vi "Report Invalid Receiver.vi"(8 "Error In":errorcluster, 10 "Receiver":string, 11 "Central Message Handler In":refnum<class "Central Message Handler.lvclass">) -> (0 "Error Out":errorcluster, 3 "Central Message Handler Out":refnum<class "Central Message Handler.lvclass">)   [LabVIEW 2019, in "Central Message Handler.lvclass"]
uses:
  Central Message Handler.lvclass
  Process/Public/Controls/Process Message.ctl
  <vilib>/Utility/error.llb/Error Cluster From Error Code.vi
  <vilib>/ErrorRing/Error Ring.xnode
  Process/Process.lvclass
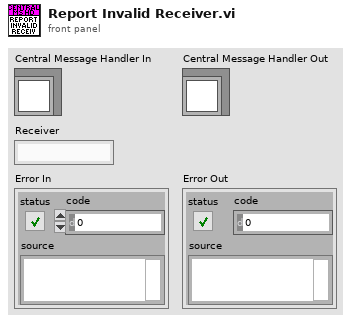
[diagram p1: front panel]
types:
  T1 = typedef "Process.lvclass/Process Message.ctl" = cluster{"Command":string, "Data":variant}
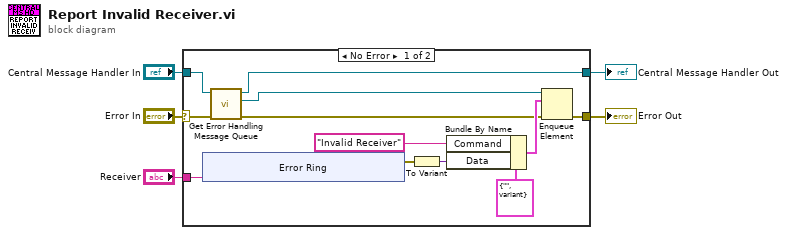
[diagram p0: block diagram]
diagram:
  n1 = case shown="No Error" "Error In" {
    selector: "Error In" -> [w10 w25]
    tunnel: "Receiver" -> [w17 _]
    tunnel: [w16 w25] -> w4
    tunnel: "Central Message Handler In" -> [w11 w26]
    tunnel: [w8 w26] -> w1
    frame No Error {
      n2 = xnode "Error Ring"("parameter 0"=w17) -> ("error out"=w6:errorcluster)
      n3 = call "Get Error Handling Message Queue.vi"("Error In"=w10, "Central Message Handler In"=w11) -> ("Error Out"=w9:errorcluster, "Error Handling Message Queue"=w14:refnum<queue>, "Central Message Handler Out"=w8:refnum<class "Central Message Handler.lvclass">)  [unwired: 7 in]
      n4 = To Variant(anything=w6) -> (Variant=w7:variant)
      n5 = Bundle By Name(cluster=T1 {"Command"="", "Data"=variant} ("element"), "Command"="Invalid Receiver", "Data"=w7) -> (w15:T1)
      n6 = Enqueue Element(queue=w14, element=w15, error in (no error)=w9) -> (error out=w16:errorcluster)  [unwired: 1 in, 2 out]
    }
    frame Error {
    }
  }
  "Error Out" <- w4
  "Central Message Handler Out" <- w1
